vi "Test Enabled Image.vi"() -> ()   [LabVIEW 2015]
panel:
  in  "coordinate space":bool
  in  "OK Button":bool
  in  "Enabled/Disabled":bool
  in  "script path":string="C:\\Users\\tilin\\Desktop\\Vision_20160307\\Data\\CCC"
  in  "stop":bool
  out "data string":string
  # "<- Run之前要改"
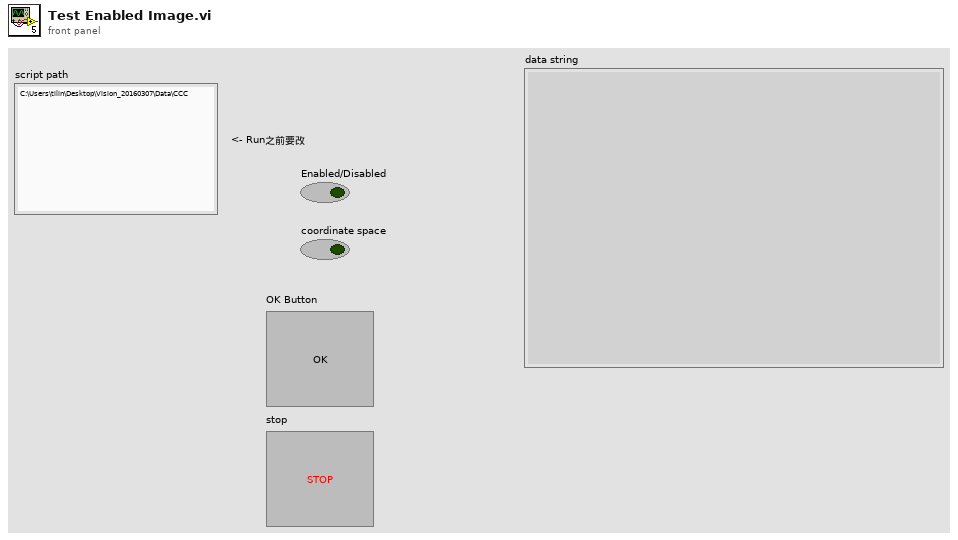
[diagram p1: front panel]
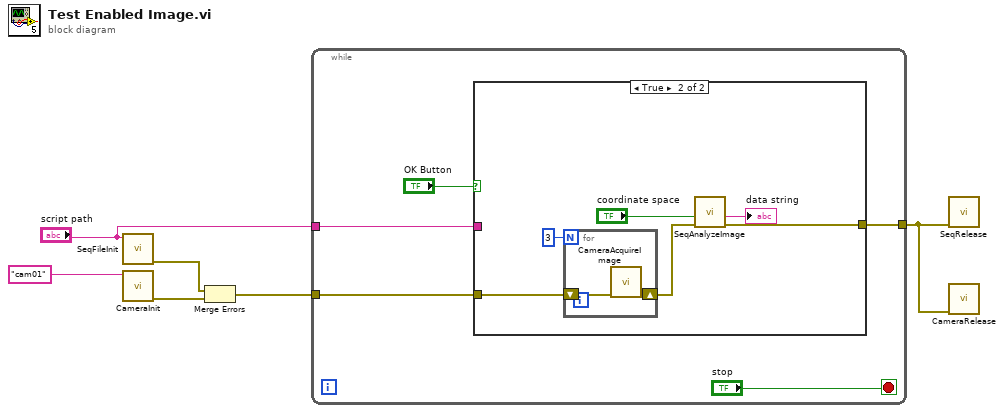
[diagram p0: block diagram]
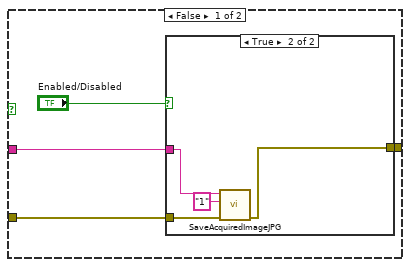
[diagram p2: hidden frame]
diagram:
  n1 = call "SeqFileInit.vi"("script path"="script path") -> ("error out"=w3:errorcluster)  [unwired: 9 in, 1 out]
  n2 = call "CameraInit.vi"("CameraName"="cam01") -> ("error out"=w5:errorcluster)  [unwired: 9 in, 1 out]
  n3 = Merge Errors(w3, w5) -> (w4:errorcluster)
  n4 = while {
    tunnel: w4 -> [w10]
    tunnel: [w9] -> w2
    tunnel: "script path" -> [w8]
    stop <- "stop" stop-if-true
    n5 = case shown="True" "OK Button" {
      tunnel: w10 -> [w14 w26]
      tunnel: [w13 w24] -> w9
      tunnel: w8 -> [w12 _]
      frame False {
        n6 = case shown="True" "Enabled/Disabled" {
          tunnel: w14 -> [w16 w20]
          tunnel: [w16 w19] -> w13
          tunnel: w12 -> [_ w18]
          frame False {
          }
          frame True {
            n7 = call "SaveAcquiredImageJPG.vi"("error in"=w20, "File Name"="1", "Folder Path"=w18) -> ("error out"=w19:errorcluster)  [unwired: 5 in, 3 out]
          }
        }
      }
      frame True {
        n8 = for {
          N: 3 -> [_]
          shift-right: [w27] -> w25
          shift-left: w26 -> [w28]
          n9 = call "CameraAcquireImage.vi"("error in"=w28) -> ("error out"=w27:errorcluster)  [unwired: 9 in, 1 out]
        }
        n10 = call "SeqAnalyzeImage.vi"("error in"=w25, "coordinate space"="coordinate space") -> ("error out"=w24:errorcluster, "data string"=→"data string":string)  [unwired: 5 in, 3 out]
      }
    }
  }
  n11 = call "SeqRelease.vi"("error in"=w2) -> ()  [unwired: 9 in, 2 out]
  n12 = call "CameraRelease.vi"("error in"=w2) -> ()  [unwired: 9 in, 2 out]
